vi "Start measurements.vi"(6 "Syncronize measurements":bool=TRUE, 8 "error in (no error)":errorcluster, 9 "Repeat times":i32=-1, 10 "Measurements":string[](array[string]), 11 "Mag Lab Measure Controller in":refnum<class "Mag Lab Measure Controller.lvclass">) -> (0 "error out":errorcluster, 3 "Mag Lab Measure Controller out":refnum<class "Mag Lab Measure Controller.lvclass">)   [LabVIEW 2015, in "Mag Lab Measure Controller.lvclass"]
uses:
  Mag Lab Measure Controller.lvclass
  Compound Measurement/Compound Measurement.lvclass/Compound Measurement.ctl
  Mag Lab Measurement/Mag Lab Measurement.lvclass/Mag Lab Measurement.ctl
  Mag Lab Root/Mag Lab Root.lvclass/Mag Lab Root.ctl
  Compound Measurement/Compound Measurement.lvclass
  Mag Lab Root/Mag Lab Root.lvclass
  Mag Lab Error Handler/Mag Lab Error Handler.lvclass
  Mag Lab Measurement/Mag Lab Measurement.lvclass
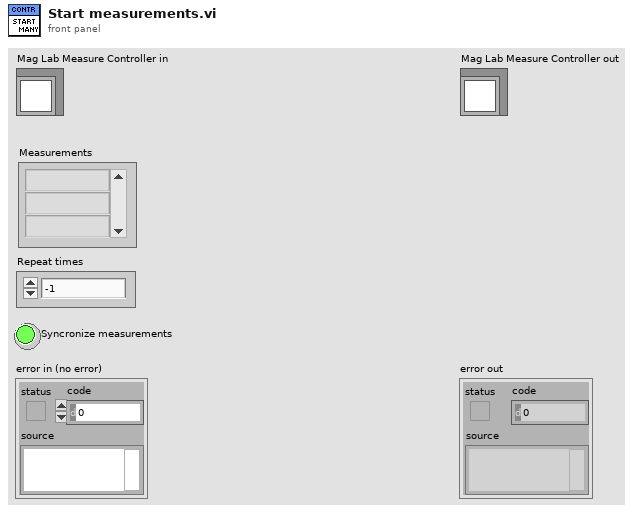
[diagram p1: front panel]
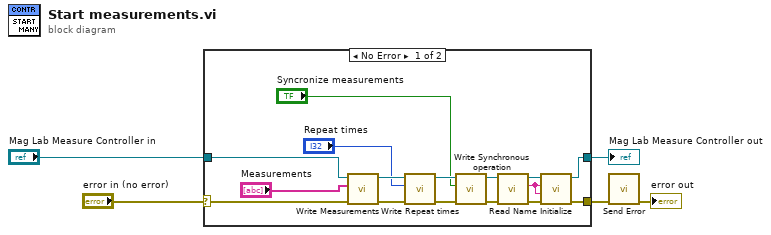
[diagram p0: block diagram]
diagram:
  n1 = case shown="No Error" "error in (no error)" {
    selector: "error in (no error)" -> [w19 w23]
    tunnel: [w17 w23] -> w2
    tunnel: [w18 w22] -> w3
    tunnel: "Mag Lab Measure Controller in" -> [w20 w22]
    frame No Error {
      n2 = call "Write Measurements.vi"("error in (no error)"=w19, "Measurements"="Measurements", "Compound Measurement in"=w20) -> ("error out"=w12:errorcluster, "Compound Measurement out"=w13:refnum<class "Mag Lab Measure Controller.lvclass">)  [unwired: 7 in]
      n3 = call "Write Repeat times.vi"("error in (no error)"=w12, "Repeat times"="Repeat times", "Mag Lab Measurement in"=w13) -> ("error out"=w10:errorcluster, "Mag Lab Measurement out"=w9:refnum<class "Mag Lab Measure Controller.lvclass">)  [unwired: 7 in]
      n4 = call "Write Synchronous operation.vi"("error in (no error)"=w10, "Synchronous operation"="Syncronize measurements", "Mag Lab Root in"=w9) -> ("error out"=w7:errorcluster, "Mag Lab Root out"=w8:refnum<class "Mag Lab Measure Controller.lvclass">)  [unwired: 7 in]
      n5 = call "Read Name.vi"("error in (no error)"=w7, "Mag Lab Root in"=w8) -> ("error out"=w15:errorcluster, "Name"=w14:string, "Mag Lab Root out"=w16:refnum<class "Mag Lab Measure Controller.lvclass">)  [unwired: 7 in]
      n6 = call-dynamic "Initialize.vi"("error in (no error)"=w15, "Requestor"=w14, "Requestee"=w14, "Mag Lab Measure Controller in"=w16) -> ("error out"=w17:errorcluster, "Mag Lab Measure Controller out"=w18:refnum<class "Mag Lab Measure Controller.lvclass">)  [unwired: 6 in]
    }
    frame Error {
    }
  }
  "Mag Lab Measure Controller out" <- w3
  n7 = call "Send Error.vi"("error in (no error)"=w2) -> ("error out"=→"error out":errorcluster)  [unwired: 9 in, 1 out]
